vi "about-clusters.vi"() -> ()   [LabVIEW 2022 SP3]
panel:
  in  "a":i32
  in  "b":bool
  in  "Tab Control":enum32{"Page 1", "Page 2", "Page 3"}(tab)
  out "Waveform Chart":dbl(graph)
  out "Waveform Graph":dbl[](graph)
  out "XY Graph":cluster{"Y":dbl[], "Y":dbl[]}[](graph)
  in  "[ESC]":bool
  out "error constant":errorcluster={"status"=FALSE, "code"=0, "source"="Everything works\njust fine!"}
  out "Out Array":dbl[](array[numeric])
  out "Out":cluster{"a":dbl, "b":bool}
  in  "In":cluster{"a":i32, "b":bool}
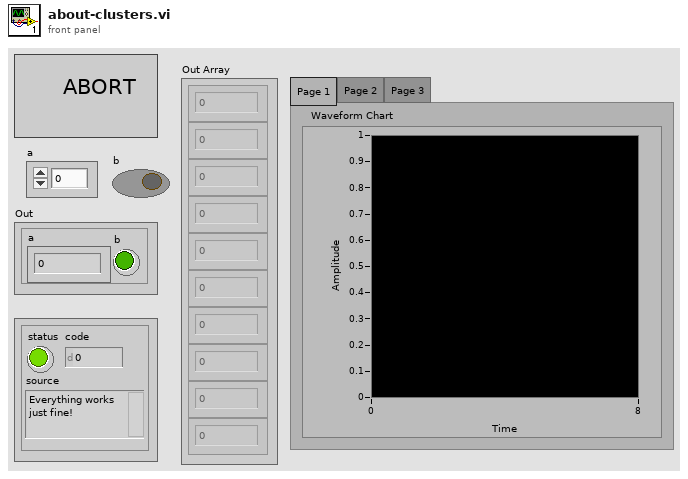
[diagram p1: front panel]
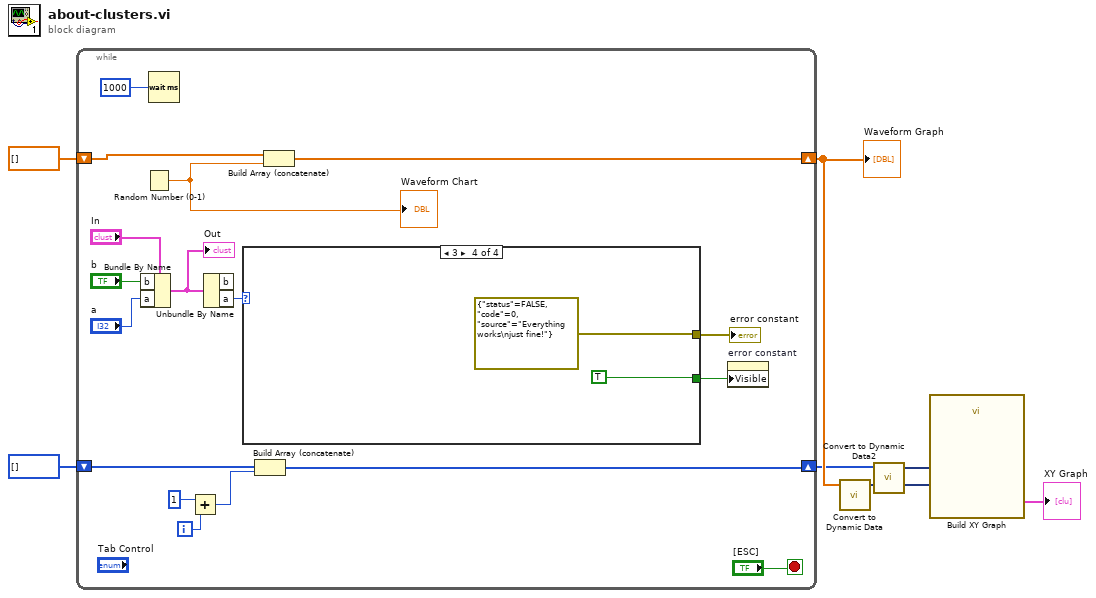
[diagram p0: block diagram]
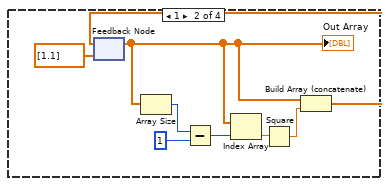
[diagram p3: hidden frame]
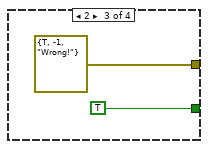
[diagram p4: hidden frame]
diagram:
  n1 = while {
    shift-right: [w23] -> w5
    shift-left: dbl[] [] -> [w22]
    shift-right: [w18] -> w3
    shift-left: i32[] [] -> [w19]
    i -> [w21]
    stop <- "[ESC]" stop-if-true
    n2 = Bundle By Name(cluster="In", "b"="b", "a"="a") -> (w14:cluster{"a":i32, "b":bool})
    "Out" <- w14
    n3 = Random Number (0-1)() -> (number: 0 to 1=w17:dbl)
    "Waveform Chart" <- w17
    n4 = Wait (ms)(milliseconds to wait=u32 1000) -> ()  [unwired: 1 out]
    n5 = Add(x=1, y=w21) -> (x+y=w16:i32)
    n6 = Unbundle By Name(w14) -> ("a"=w13:i32)  [unwired: 1 out]
    n7 = case shown="3" w13 {
      tunnel: [_ _ errorcluster {"status"=TRUE, "code"=-1, "source"="Wrong!"} ("error constant") errorcluster {"status"=FALSE, "code"=0, "source"="Everything works\njust fine!"} ("error constant")] -> w8
      tunnel: [_ _ TRUE ("Visible") TRUE ("Visible")] -> w9
      frame 0, Default {
      }
      frame 1 {
        n8 = feedback #1(dbl[] [1.1]) -> (w25:dbl[])
        "Out Array" <- w25
        n9 = Array Size(array=w25) -> (size(s)=w27:i32)
        n10 = Subtract(x=w27, y=1) -> (x-y=w26:i32)
        n11 = Index Array(array=w25, index=w26) -> (element=w31:dbl)
        n12 = Square(x=w31) -> (x^2=w32:dbl)
        n13 = Build Array (concatenate)(w25, w32) -> (w30:dbl[])
        n14 = feedback-in #1(w30) -> ()
      }
      frame 2 {
      }
      frame 3 {
      }
    }
    "error constant" <- w8
    n15 = Build Array (concatenate)(w19, w16) -> (w18:i32[])
    n16 = Build Array (concatenate)(w22, w17) -> (w23:dbl[])
    n17 = property on="error constant" class="Clust (strict)"("Visible"=w9) -> ()  [unwired: 2 in, 2 out]
  }
  "Waveform Graph" <- w5
  n18 = call "Convert to Dynamic Data"("Array"=w5) -> ("Dynamic Data Type"=w4:dynamicdata)  [unwired: 3 in]
  n19 = call "Convert to Dynamic Data2"("Array"=w3) -> ("Dynamic Data Type"=w2:dynamicdata)  [unwired: 3 in]
  n20 = call "Build XY Graph"("Y Input"=w4, "X Input"=w2) -> ("XY Graph"=→"XY Graph":cluster{"Y":dbl[], "Y":dbl[]}[])  [unwired: 3 in, 6 out]
